vi "09 Clusters.vi"() -> ()   [LabVIEW 2019]
uses:
  _Subs/OpenDiagram/Open_XControl.xctl
panel:
  in  "OpenDiag":refnum<vi>(xcontrol)
  out "Waveform Graph":T1(graph)
  out "Clusters and Plots 2":cluster{i32, "number: 0 to 1":dbl}[](graph)
  out "Clusters and Plots":cluster{i32[], dbl[]}(graph)
  out "Add 10 to height and\nnegate attendance":T2
  out "Add Dr. to name and \nchange height":T2
  in  "Cluster":T2={"Name"="Al Einstein", "Height (cm)"=170.0, "attended"=FALSE}
  # "09 Clusters\nThis code demonstrates some ways of using clusters (similar to structures in other languages). \nA cluster is a grouping of data elements of any type.  \n\nInstructions:\n1. Open the block diagram and read the descriptions. \n2. Hit the Run arrow and see the code run. Modify cluster inputs to see how outputs change."
  # "Right click to change \nautomatic arrangement"
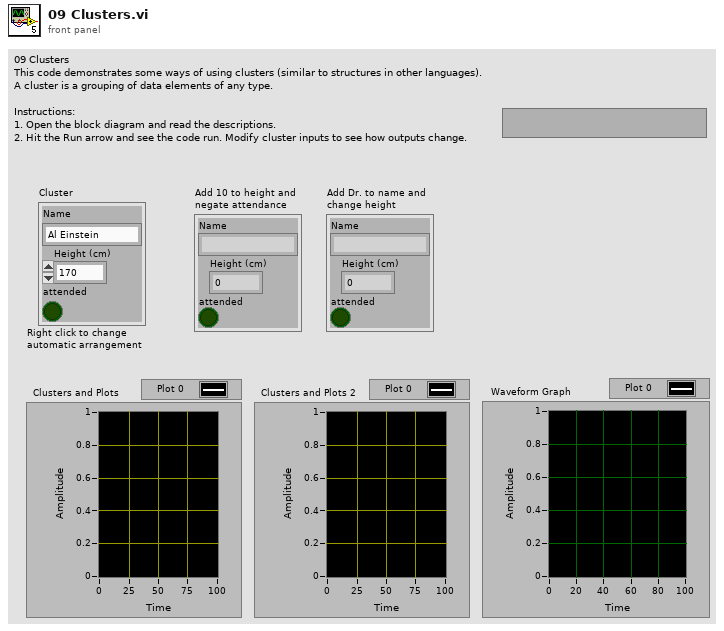
[diagram p1: front panel]
types:
  T1 = cluster{"Height (cm)":dbl, "Height (cm)":dbl, dbl[]}
  T2 = cluster{"Name":string, "Height (cm)":dbl, "attended":bool}
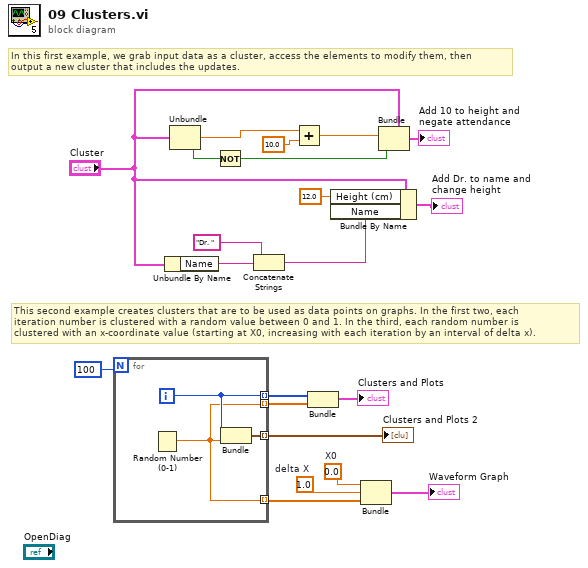
[diagram p0: block diagram]
diagram:
  w1 = 1.0  # delta X
  w2 = 0.0  # X0
  # "This second example creates clusters that are to be used as data points on graphs. In the first two, each\niteration number is clustered with a random value between 0 and 1. In the third, each random number is \nclustered with an x-coordinate value (starting at X0, increasing with each iteration by an interval of delta x)."
  # "In this first example, we grab input data as a cluster, access the elements to modify them, then \noutput a new cluster that includes the updates."
  n1 = for {
    N: 100 -> [_]
    tunnel: [w24] -> w9 mode=indexing
    tunnel: [w22] -> w8 mode=indexing
    tunnel: [w23] -> w5 mode=indexing
    tunnel: [w22] -> w4 mode=indexing
    i -> [w24]
    n2 = Random Number (0-1)() -> (number: 0 to 1=w22:dbl)
    n3 = Bundle(w24, "number: 0 to 1"=w22) -> (w23:cluster{i32, "number: 0 to 1":dbl})  [unwired: 1 in]
  }
  "Clusters and Plots 2" <- w5
  n4 = Unbundle By Name("Cluster") -> ("Name"=w12:string)
  n5 = Unbundle("Cluster") -> ("Height (cm)"=w18:dbl, "attended"=w15:bool)  [unwired: 1 out]
  n6 = Not(x=w15) -> (.not. x?=w14:bool)
  n7 = Concatenate Strings("Dr. " ("string"), w12) -> (w10:string)
  n8 = Add(x=w18, y=10.0) -> (x+y=w16:dbl)
  n9 = Bundle(w9, w8) -> (→"Clusters and Plots":cluster{i32[], dbl[]})  [unwired: 1 in]
  n10 = Bundle By Name(cluster="Cluster", "Height (cm)"=12.0, "Name"=w10) -> (→"Add Dr. to name and \nchange height":T2)
  n11 = Bundle("X0"=w2, "delta X"=w1, w4) -> (→"Waveform Graph":cluster{"X0":dbl, "delta X":dbl, dbl[]})  [unwired: 1 in]
  n12 = Bundle(cluster="Cluster", "Height (cm)"=w16, "attended"=w14) -> (→"Add 10 to height and\nnegate attendance":T2)  [unwired: 1 in]
